vi "ValveMonitoring.vi"() -> ()   [LabVIEW 2020]
uses:
  Control/MainProgramState.ctl
  <vilib>/DAQmx/read.llb/DAQmx Read (Analog 1D DBL NChan 1Samp).vi
  <vilib>/DAQmx/create/channels.llb/DAQmx Create Channel (AI-Voltage-Basic).vi
  <vilib>/DAQmx/miscellaneous.llb/DAQmx Fill In Error Info.vi
  <resource>/objmgr/daqmx.rc
panel:
  out "RemainTime":dbl(slide) scale=0.0..1.0
  in  "TermiateTime(min)":dbl=60.0 format="%.1f"
  out "FlowRate(Average)":dbl format="%.3f"
  out "ProgramState":T1
  out "Active":bool
  in  "Set":bool
  out "TestTimer(sec)":dbl format="%.1f"
  out "SystemTimer(sec)":dbl format="%.1f"
  out "FlowRate":dbl format="%.3f"
  out "Pressure":dbl format="%.1f"
  out "TestTimer(min)":dbl
  out "FlowRateLowWarning":bool
  in  "FlowRateUpperLimit(LPM)":dbl=1.0 format="%.3f"
  in  "PressureLowerLimit(bar)":dbl=5.0 format="%.1f"
  out "PressureLowWarning":bool
  in  "Reset":bool
  out "SystemTimer(min)":dbl
  in  "FileName":string="Test"
  in  "Stop":bool
  in  "Pause":bool
  in  "Start":bool
  out "StopSignal":bool
  out "appended array":dbl[](array[numeric])
  out "FlowRate":cluster{dbl[], dbl[]}(graph)
  out "Pressure":cluster{dbl[], dbl[]}(graph)
  # "Test Setting"
  # "<- Logging Fine Name"
  # "Program State"
  # "System Timer"
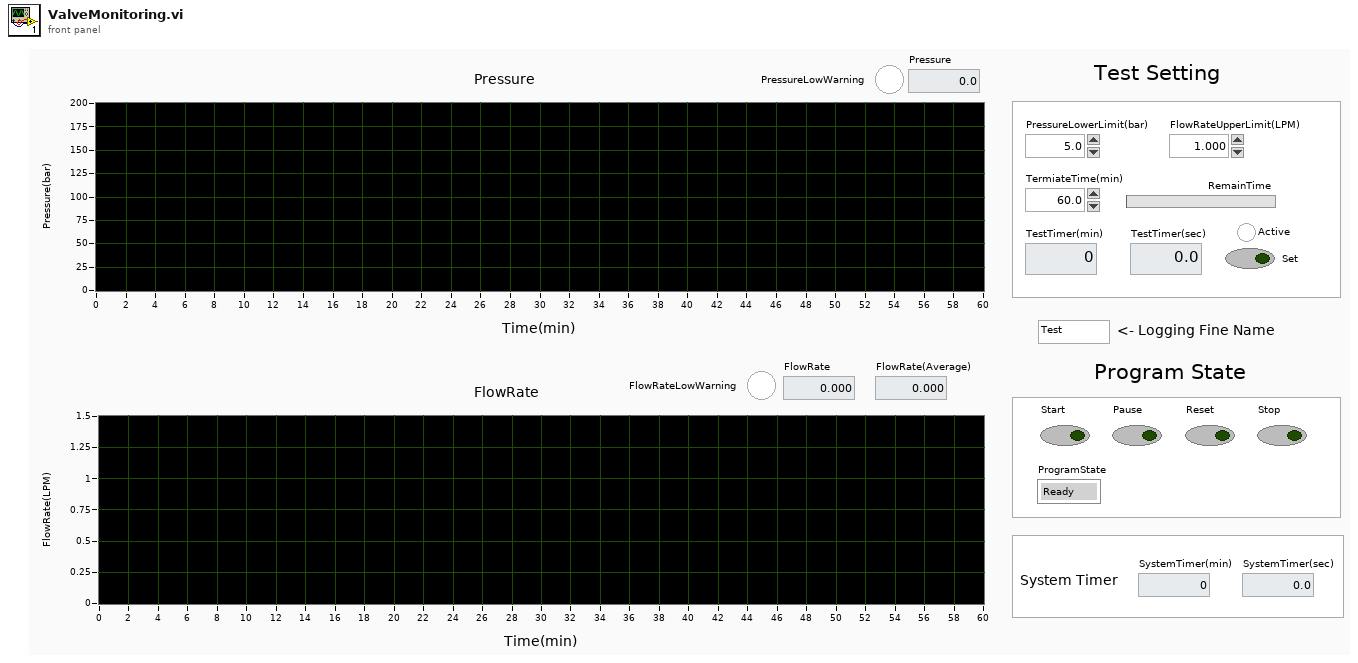
[diagram p1: front panel]
types:
  T1 = typedef "MainProgramState.ctl" = enum16{"Ready", "Run", "Pause", "Reset", "Stop"}
  T2 = cluster{"State":T1, "MainTimer(sec)":dbl, "TestTimer(sec)":dbl}
  T3 = enum16{"open", "replace", "create", "open or create", "replace or create", "replace or create with confirmation"}
  T4 = cluster{"getFlowRate":dbl, "getPressure":dbl, "setFlowRate":dbl, "setPressure":dbl}
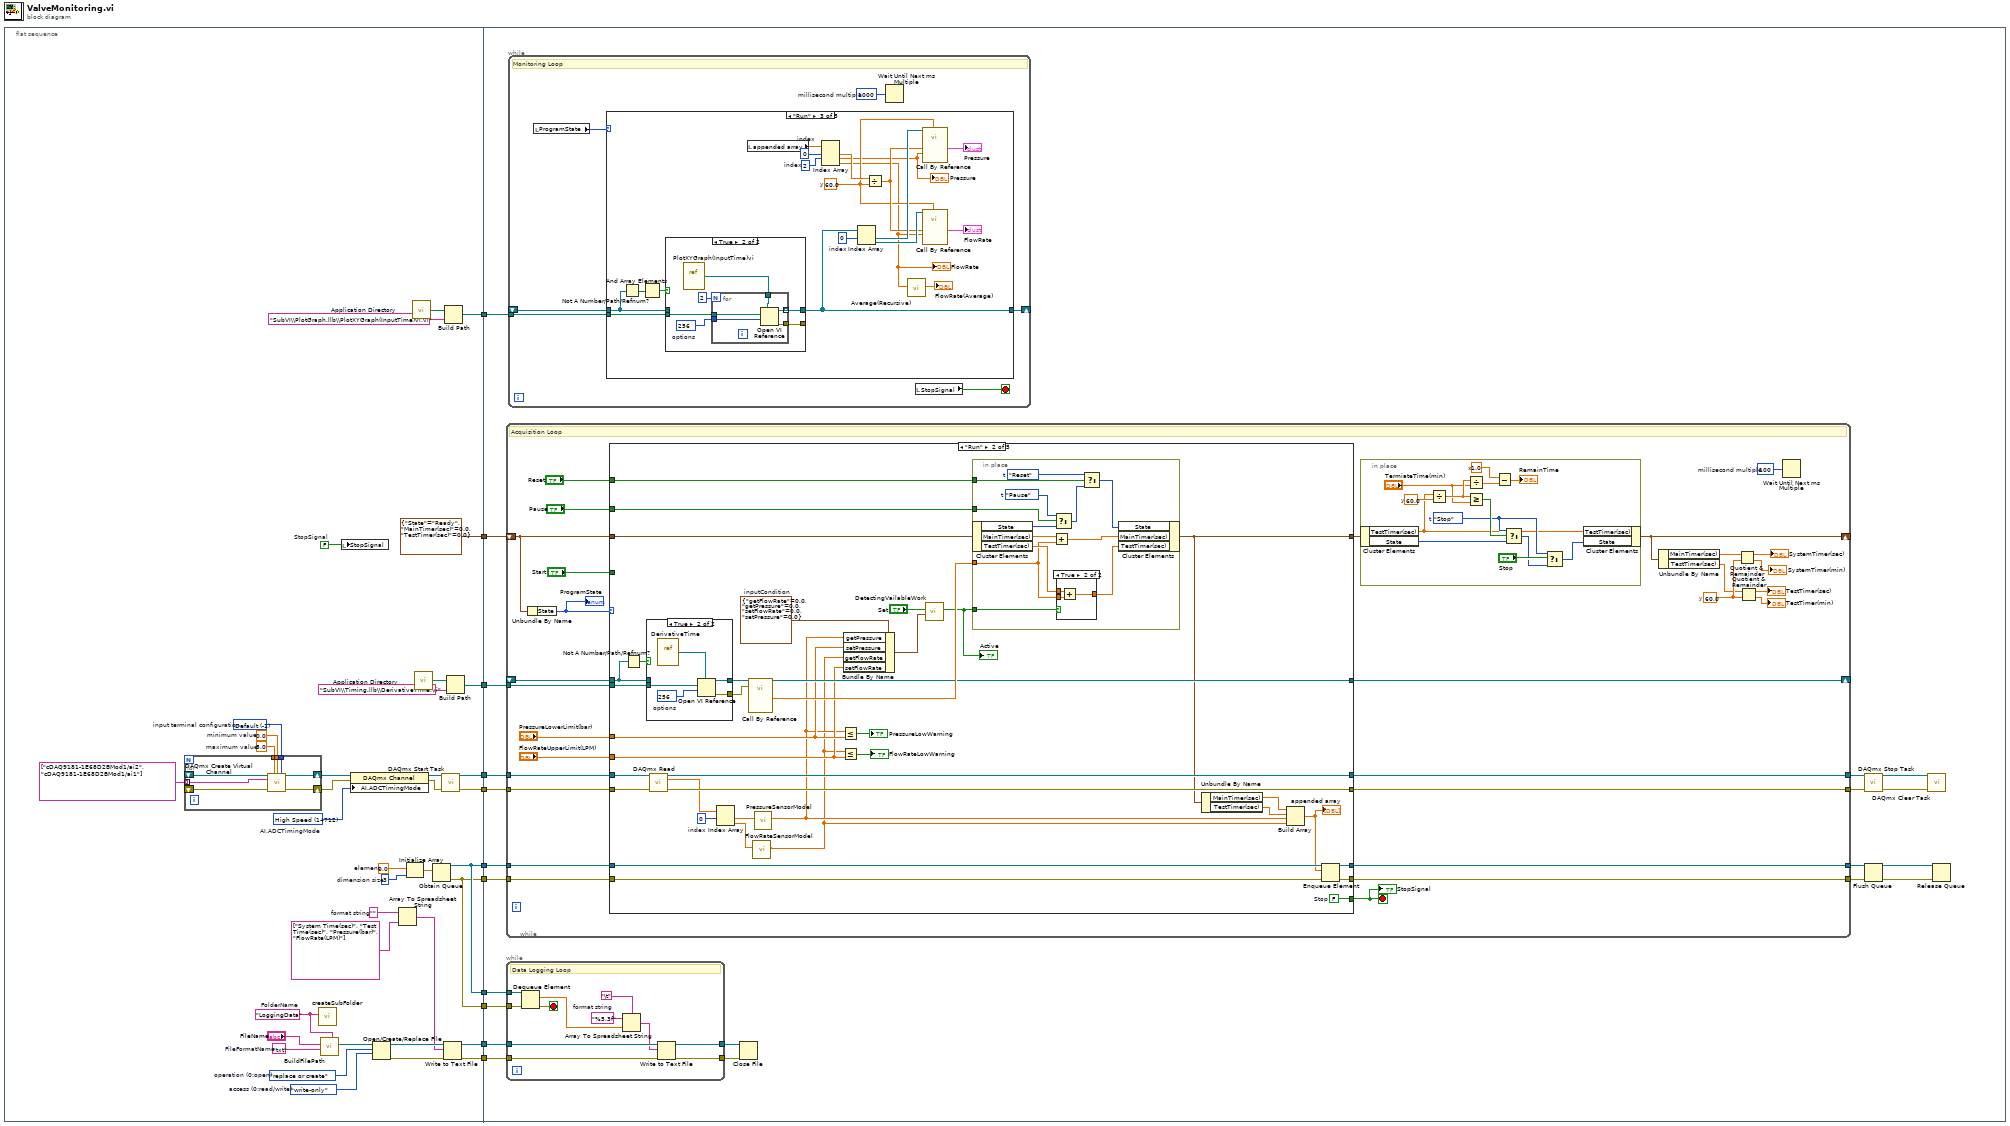
[diagram p0: block diagram]
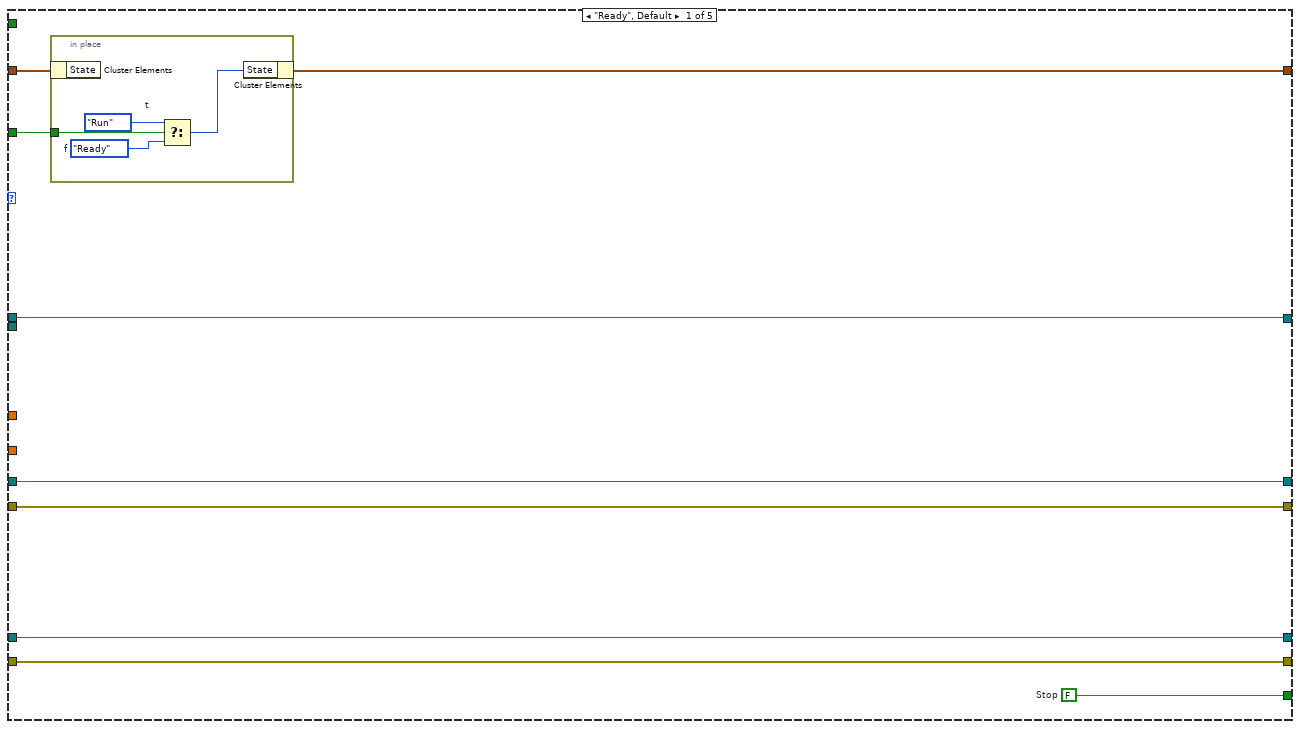
[diagram p2: hidden frame]
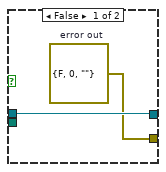
[diagram p3: hidden frame]
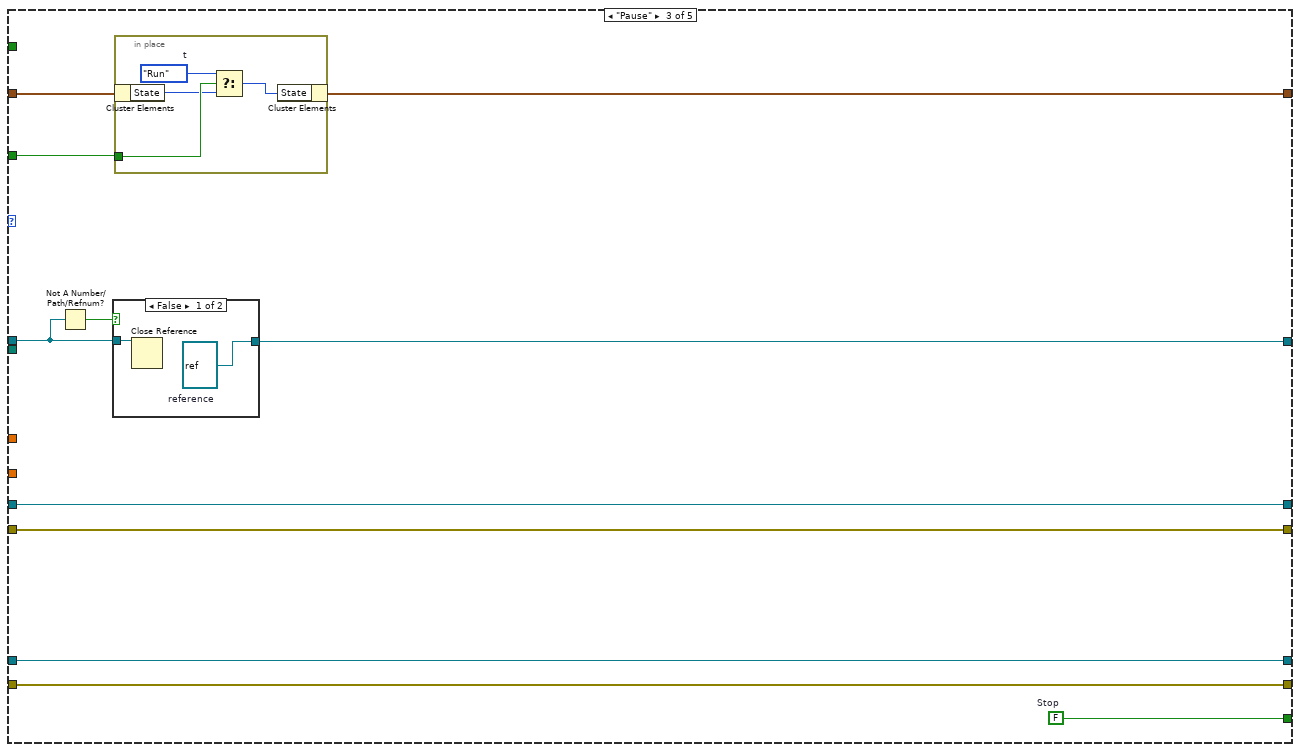
[diagram p5: hidden frame]
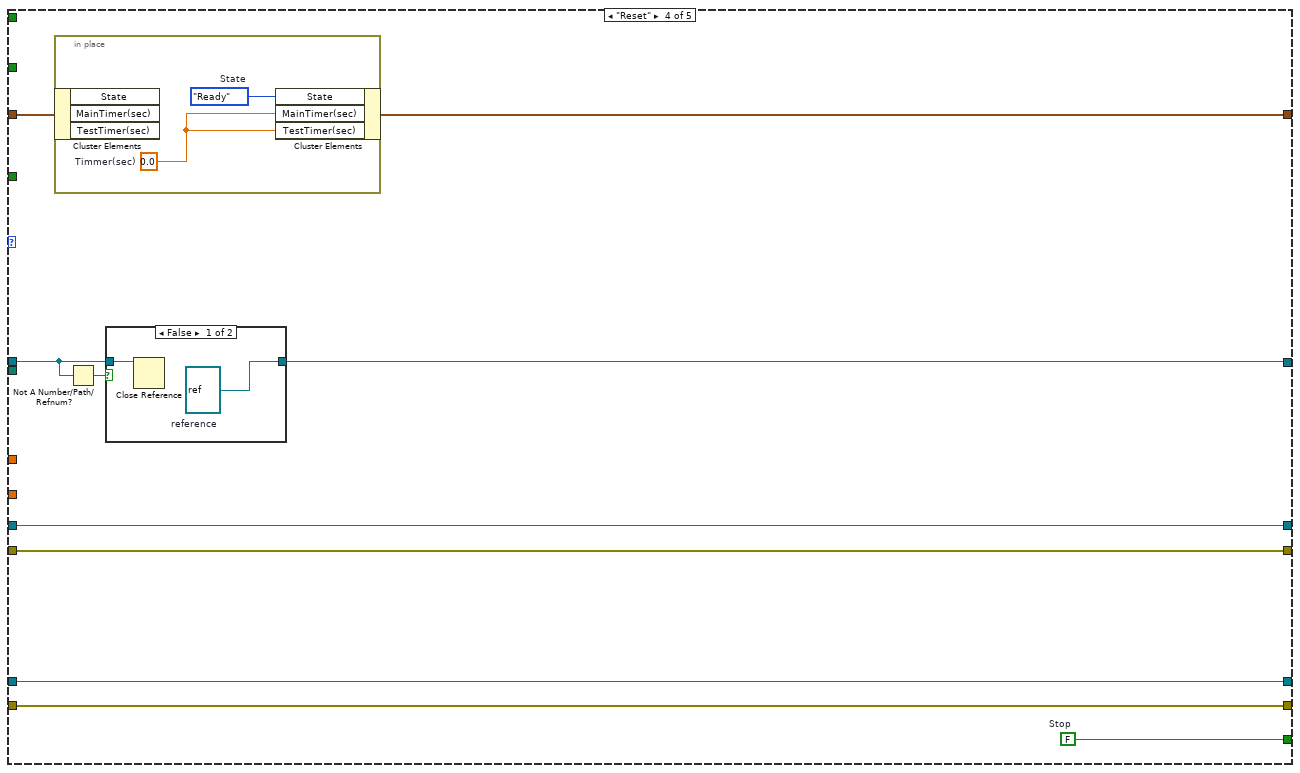
[diagram p7: hidden frame]
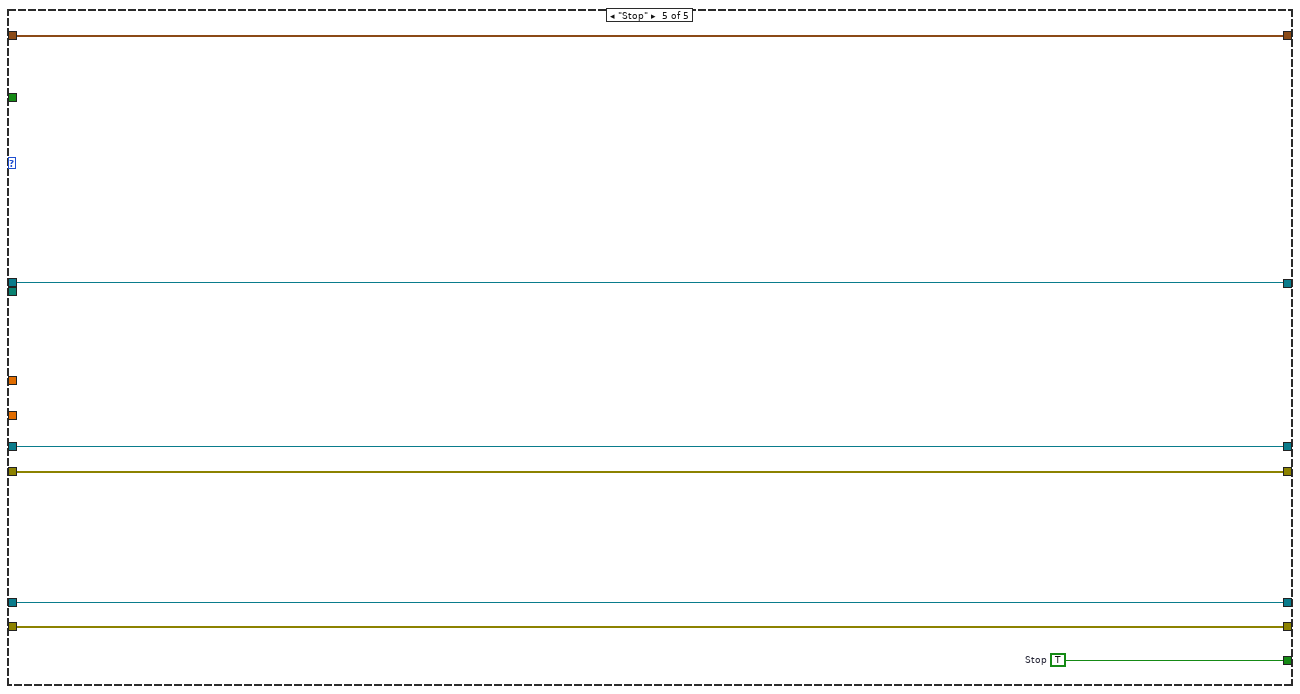
[diagram p9: hidden frame]
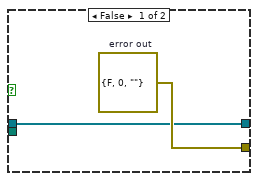
[diagram p12: hidden frame]
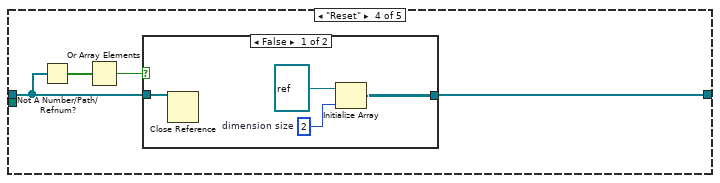
[diagram p13: hidden frame]
diagram:
  n1 = flat-sequence {
    tunnel: [w36] -> w11
    tunnel: [w35] -> w10
    tunnel: [w43] -> w9
    tunnel: [w42] -> w8
    tunnel: [w43] -> w7
    tunnel: [w42] -> w6
    tunnel: [w32] -> w5
    tunnel: [w31] -> w4
    tunnel: [T2 {"State"=enum."Ready", "MainTimer(sec)"=0.0, "TestTimer(sec)"=0.0}] -> w3
    tunnel: [w16] -> w2
    tunnel: [w12] -> w1
    tunnel: w11 -> [w77]
    tunnel: w10 -> [w72]
    tunnel: w9 -> [w71]
    tunnel: w8 -> [w70]
    tunnel: w7 -> [w65]
    tunnel: w6 -> [w64]
    tunnel: w5 -> [w63]
    tunnel: w4 -> [w62]
    tunnel: w3 -> [w59]
    tunnel: w2 -> [w58]
    tunnel: w1 -> [w57]
    frame #0 {
      w18 = FALSE  # StopSignal
      w19 = 14712 items=["Automatic"=16097, "High Resolution"=10195, "High Speed"=14712, "Best 50 Hz Rejection"=14713, "Best 60 Hz Rejection"=14714, "Custom"=10137]  # AI.ADCTimingMode
      w25 = "txt"  # FileFormatName
      w28 = ""  # format string
      w37 = enum16{"read/write", "read-only", "write-only"}."write-only"  # access (0:read/write)
      w38 = T3."replace or create"  # operation (0:open)
      w40 = "LoggingData"  # FolderName
      w41 = -1 items=["Default"=-1, "RSE"=10083, "NRSE"=10078, "Differential"=10106, "Pseudodifferential"=12529]  # input terminal configuration
      w45 = 3  # dimension size
      w46 = 0.0  # element
      w47 = 0.0  # minimum value
      w48 = 5.0  # maximum value
      n2 = for {
        tunnel: w48 -> [w56]
        tunnel: w47 -> [w55]
        tunnel: w41 -> [w54]
        shift-right: [w53] -> w24
        shift-left: _ -> [w52]
        tunnel: tag[] ["cDAQ9181-1E68D2BMod1/ai2", "cDAQ9181-1E68D2BMod1/ai1"] -> [w51] mode=indexing
        shift-right: [w50] -> w21
        shift-left: _ -> [w49]
        n3 = call-poly <vilib>:"DAQmx Create Virtual Channel.vi"("task in"=w52, "maximum value"=w56, "minimum value"=w55, "input terminal configuration"=w54, "physical channels"=w51, "error in"=w49) -> ("task out"=w53:refnum<k21>, "error out"=w50:errorcluster)  [unwired: 8 in]
      }
      n4 = call "createSubFolder.vi"("FolderName"=w40) -> ()  [unwired: 10 in, 1 out]
      n5 = call "BuildFilePath.vi"("SubFolderName"=w40, "FileFormatName"=w25, "FileName"="FileName") -> ("appended path"=w39:path)  [unwired: 8 in]
      n6 = local write "StopSignal"(w18) -> ()
      n7 = property class="DAQmx Channel"(reference=w24, error in=w21, "AI.ADCTimingMode"=w19) -> (reference out=w22:refnum<k21>, error out=w20:errorcluster)
      n8 = Open/Create/Replace File(file path (use dialog)=w39, operation (0:open)=w38, access (0:read/write)=w37) -> (refnum out=w34:refnum<file>, error out=w33:errorcluster)  [unwired: 3 in, 1 out]
      n9 = Array To Spreadsheet String(array=string[] ["System Time(sec)", "Test Time(sec)", "Pressure(bar)", "FlowRate(LPM)"], 3:w28) -> (spreadsheet string=w29:string)  [unwired: 1 in]
      n10 = Initialize Array "Initialize Array"(w46, w45) -> (w44:dbl[])
      n11 = call <vilib>:"Application Directory.vi"() -> ("Application Directory"=w14:path)
      n12 = call <vilib>:"Application Directory.vi"() -> ("Application Directory"=w15:path)
      n13 = Obtain Queue(element data type=w44) -> (queue out=w43:refnum<queue>, error out=w42:errorcluster)  [unwired: 4 in, 1 out]
      n14 = call <vilib>:"DAQmx Start Task.vi"("task/channels in"=w22, "error in"=w20) -> ("task out"=w36:refnum<k21>, "error out"=w35:errorcluster)  [unwired: 12 in]
      n15 = Write to Text File(file (use dialog)=w34, text=w29, error in=w33) -> (refnum out=w32:refnum<file>, error out=w31:errorcluster)  [unwired: 1 in, 1 out]
      n16 = Build Path(base path=w14, name or relative path="SubVI\\PlotGraph.llb\\PlotXYGraph(InputTime)vi.vi") -> (appended path=w12:path)
      n17 = Build Path(base path=w15, name or relative path="SubVI\\Timing.llb\\DerivativeTime.vi") -> (appended path=w16:path)
    }
    frame #1 {
      n18 = while {
        tunnel: w77 -> [w117]
        tunnel: [w116] -> w76
        tunnel: [w115] -> w74
        tunnel: w72 -> [w114]
        tunnel: w71 -> [w113]
        tunnel: w70 -> [w112]
        tunnel: [w111] -> w69
        tunnel: [w110] -> w68
        shift-right: [w102] -> _
        shift-left: w59 -> [w104]
        tunnel: w58 -> [w101]
        shift-right: [w100] -> _
        shift-left: _ -> [w99]
        stop <- w106 stop-if-true
        w91 = 60.0  # y
        w109 = u32 100  # millisecond multiple
        # "Acquisition Loop"
        n19 = Unbundle By Name(w104) -> ("State"=w105:T1)
        "ProgramState" <- w105
        n20 = case shown="\"Run\"" w105 {
          tunnel: w117 -> [w126 w167 w202 w217 w228]
          tunnel: [w126 w166 w202 w217 w228] -> w116
          tunnel: [w125 w165 w201 w216 w227] -> w115
          tunnel: w114 -> [w125 w164 w201 w216 w227]
          tunnel: w113 -> [w124 w163 w200 w215 w230]
          tunnel: w112 -> [w123 w162 w199 w214 w229]
          tunnel: [w124 w161 w200 w215 w230] -> w111
          tunnel: [w123 w160 w199 w214 w229] -> w110
          tunnel: "Start" -> [w119 _ w195 _ _]
          tunnel: "Pause" -> [_ w157 _ _ _]
          tunnel: [w122 w159 w198 w213 w231] -> w106
          tunnel: [w120 w133 w196 w218 w226] -> w103
          tunnel: w104 -> [w121 w153 w197 w219 w226]
          tunnel: w101 -> [_ w154 _ _ _]
          tunnel: [w118 w150 w192 w210 w225] -> w100
          tunnel: w99 -> [w118 w149 w193 w211 w225]
          tunnel: "Reset" -> [_ w144 _ _ _]
          tunnel: "PressureLowerLimit(bar)" -> [_ w141 _ _ _]
          tunnel: "FlowRateUpperLimit(LPM)" -> [_ w140 _ _ _]
          frame "Ready", Default {
            w122 = FALSE  # Stop
            n21 = in-place {
              in-place-border: w119 -> [w128]
              w130 = MainProgramState."Ready"  # f
              w129 = MainProgramState."Run"  # t
              n22 = in-place-cluster #1(w121) -> ()  [unwired: 1 out]
              n23 = Select(t=w129, s=w128, f=w130) -> (s? t:f=w127:T1)
              n24 = in-place-cluster #1("State"=w127) -> (w120:T2)
            }
          }
          frame "Run" {
            w139 = T4 {"getFlowRate"=0.0, "getPressure"=0.0, "setFlowRate"=0.0, "setPressure"=0.0}  # inputCondition
            w147 = 0  # index
            w159 = FALSE  # Stop
            n25 = Not A Number/Path/Refnum?(number/path/refnum=w149) -> (NaN/Path/Refnum?=w155:bool)
            n26 = case shown="True" w155 {
              tunnel: w154 -> [_ w173]
              tunnel: [w169 w171] -> w152
              tunnel: [w168 w170] -> w151
              tunnel: w149 -> [w169 _]
              frame False {
                w168 = errorcluster {"status"=FALSE, "code"=0, "source"=""}  # error out
              }
              frame True {
                w174 = 256  # options
                n27 = vi-ref "DerivativeTime.vi"() -> (w172:refnum<vi>)
                n28 = Open VI Reference(type specifier VI Refnum (for type only)=w172, vi path=w173, options=w174) -> (vi reference=w171:refnum<vi>, error out=w170:errorcluster)  [unwired: 3 in]
              }
            }
            n29 = call-poly <vilib>:"DAQmx Read.vi"("task/channels in"=w167, "error in"=w164) -> ("task out"=w166:refnum<k21>, "data"=w148:dbl[], "error out"=w165:errorcluster)  [unwired: 11 in]
            n30 = Index Array "Index Array"(array=w148, index #1=w147) -> (element #1=w145:dbl, element #2=w146:dbl)  [unwired: 1 in]
            n31 = call-by-ref "Call By Reference"(reference=w152, error in=w151) -> (reference out=w150:refnum<vi>, "Time(sec)"=w156:dbl)  [unwired: 11 in, 1 out]
            n32 = call "FlowRateSensorModel.vi"("inputSignal(V)"=w146) -> ("FlowRate(LPM)"=w134:dbl)  [unwired: 10 in]
            n33 = call "PressureSensorModel.vi"("inputSignal(V)"=w145) -> ("Pressure(bar)"=w135:dbl)  [unwired: 10 in]
            n34 = Less Or Equal?(x=w135, y=w141) -> (x <= y?=→"PressureLowWarning":bool)
            n35 = Less Or Equal?(x=w134, y=w140) -> (x <= y?=→"FlowRateLowWarning":bool)
            n36 = Bundle By Name(cluster=w139, "getPressure"=w135, "setPressure"=w141, "getFlowRate"=w134, "setFlowRate"=w140) -> (w138:T4)
            n37 = call "DetectingVailableWork.vi"("inputCondition"=w138, "Reset"="Set") -> ("Progressing"=w137:bool)  [unwired: 9 in]
            "Active" <- w137
            n38 = in-place {
              in-place-border: w156 -> [w181]
              in-place-border: w157 -> [w184]
              in-place-border: w144 -> [w179]
              in-place-border: w137 -> [w175]
              w177 = MainProgramState."Reset"  # t
              w183 = MainProgramState."Pause"  # t
              n39 = in-place-cluster #2(w153) -> ("State"=w185:T1, "MainTimer(sec)"=w187:dbl, "TestTimer(sec)"=w182:dbl)
              n40 = Add(x=w187, y=w181) -> (x+y=w186:dbl)
              n41 = Select(t=w183, s=w184, f=w185) -> (s? t:f=w180:T1)
              n42 = case shown="True" w175 {
                tunnel: w182 -> [w188 w191]
                tunnel: w181 -> [_ w190]
                tunnel: [w188 w189] -> w176
                frame False {
                }
                frame True {
                  n43 = Add(x=w191, y=w190) -> (x+y=w189:dbl)
                }
              }
              n44 = Select(t=w177, s=w179, f=w180) -> (s? t:f=w178:T1)
              n45 = in-place-cluster #2("State"=w178, "MainTimer(sec)"=w186, "TestTimer(sec)"=w176) -> (w133:T2)
            }
            n46 = Unbundle By Name(w133) -> ("MainTimer(sec)"=w132:dbl, "TestTimer(sec)"=w131:dbl)
            n47 = Build Array "Build Array"(w132, w131, w135, w134) -> (w158:dbl[])
            "appended array" <- w158
            n48 = Enqueue Element(queue=w163, element=w158, error in (no error)=w162) -> (queue out=w161:refnum<queue>, error out=w160:errorcluster)  [unwired: 1 in, 1 out]
          }
          frame "Pause" {
            w198 = FALSE  # Stop
            n49 = Not A Number/Path/Refnum?(number/path/refnum=w193) -> (NaN/Path/Refnum?=w194:bool)
            n50 = case shown="False" w194 {
              tunnel: w193 -> [w204 w205]
              tunnel: [w203 w205] -> w192
              frame False {
                w203 = refnum<vi> refnum  # reference
                n51 = Close Reference(reference=w204) -> ()  [unwired: 1 in, 1 out]
              }
              frame True {
              }
            }
            n52 = in-place {
              in-place-border: w195 -> [w209]
              w206 = MainProgramState."Run"  # t
              n53 = in-place-cluster #3(w197) -> ("State"=w208:T1)
              n54 = Select(t=w206, s=w209, f=w208) -> (s? t:f=w207:T1)
              n55 = in-place-cluster #3("State"=w207) -> (w196:T2)
            }
          }
          frame "Reset" {
            w213 = FALSE  # Stop
            n56 = in-place {
              w224 = MainProgramState."Ready"  # State
              w223 = 0.0  # Timmer(sec)
              n57 = in-place-cluster #4(w219) -> ()  [unwired: 3 out]
              n58 = in-place-cluster #4("State"=w224, "MainTimer(sec)"=w223, "TestTimer(sec)"=w223) -> (w218:T2)
            }
            n59 = Not A Number/Path/Refnum?(number/path/refnum=w211) -> (NaN/Path/Refnum?=w212:bool)
            n60 = case shown="False" w212 {
              tunnel: w211 -> [w221 w222]
              tunnel: [w220 w222] -> w210
              frame False {
                w220 = refnum<vi> refnum  # reference
                n61 = Close Reference(reference=w221) -> ()  [unwired: 1 in, 1 out]
              }
              frame True {
              }
            }
          }
          frame "Stop" {
            w231 = TRUE  # Stop
          }
        }
        "StopSignal" <- w106
        n62 = in-place {
          w233 = 1.0  # x
          w243 = 60.0  # y
          w239 = MainProgramState."Stop"  # t
          n63 = in-place-cluster #5(w103) -> ("TestTimer(sec)"=w237:dbl, "State"=w241:T1)
          n64 = Divide(x=w237, y=w243) -> (x/y=w236:dbl)
          n65 = Divide(x=w236, y="TermiateTime(min)") -> (x/y=w234:dbl)
          n66 = Greater Or Equal?(x=w236, y="TermiateTime(min)") -> (x >= y?=w242:bool)
          n67 = Subtract(x=w233, y=w234) -> (x-y=→"RemainTime":dbl)
          n68 = Select(t=w239, s=w242, f=w241) -> (s? t:f=w240:T1)
          n69 = Select(t=w239, s="Stop", f=w240) -> (s? t:f=w238:T1)
          n70 = in-place-cluster #5("TestTimer(sec)"=w237, "State"=w238) -> (w102:T2)
        }
        n71 = Unbundle By Name(w102) -> ("MainTimer(sec)"=w95:dbl, "TestTimer(sec)"=w90:dbl)
        n72 = Quotient & Remainder(x=w95, y=w91) -> (x-y*floor(x/y)=→"SystemTimer(sec)":dbl, floor(x/y)=→"SystemTimer(min)":dbl)
        n73 = Quotient & Remainder(x=w90, y=w91) -> (x-y*floor(x/y)=→"TestTimer(sec)":dbl, floor(x/y)=→"TestTimer(min)":dbl)
        n74 = Wait Until Next ms Multiple(millisecond multiple=w109) -> ()  [unwired: 1 out]
      }
      n75 = while {
        tunnel: w65 -> [w88]
        tunnel: w64 -> [w87]
        tunnel: w63 -> [w85]
        tunnel: w62 -> [w80]
        tunnel: [w79] -> w61
        tunnel: [w78] -> w60
        stop <- w86 stop-if-true
        w83 = "%5.3f"  # format string
        # "Data Logging Loop"
        n76 = Dequeue Element(queue=w88, error in (no error)=w87) -> (element=w82:dbl[], error out=w86:errorcluster)  [unwired: 1 in, 2 out]
        n77 = Array To Spreadsheet String(delimiter (Tab)="\t", array=w82, 3:w83) -> (spreadsheet string=w81:string)
        n78 = Write to Text File(file (use dialog)=w85, text=w81, error in=w80) -> (refnum out=w79:refnum<file>, error out=w78:errorcluster)  [unwired: 1 in, 1 out]
      }
      n79 = while {
        tunnel: w57 -> [w247]
        shift-right: [w246] -> _
        shift-left: _ -> [w245]
        stop <- w249 stop-if-true
        w250 = u32 1000  # millisecond multiple
        # "Monitoring Loop"
        n80 = local read "ProgramState"() -> (w248:T1)
        n81 = case shown="\"Run\"" w248 {
          tunnel: w247 -> [_ _ w268 _ _]
          tunnel: [w251 w252 w266 w285 w294] -> w246
          tunnel: w245 -> [w251 w252 w263 w287 w294]
          frame "Ready", Default {
          }
          frame "Pause" {
          }
          frame "Run" {
            w255 = 2  # index
            w267 = 0  # index
            w257 = 60.0  # y
            w270 = 0  # index
            n82 = Not A Number/Path/Refnum?(number/path/refnum=w263) -> (NaN/Path/Refnum?=w265:bool[])
            n83 = And Array Elements(Boolean array=w265) -> (logical AND=w264:bool)
            n84 = case shown="True" w264 {
              tunnel: w268 -> [_ w278]
              tunnel: [w272 w276] -> w266
              tunnel: [w273 w275] -> _
              tunnel: w263 -> [w272 _]
              frame False {
                w273 = errorcluster {"status"=FALSE, "code"=0, "source"=""}  # error out
              }
              frame True {
                w279 = 256  # options
                n85 = vi-ref "PlotXYGraph(InputTime)vi.vi"() -> (w277:refnum<vi>)
                n86 = for {
                  N: 2 -> [_]
                  tunnel: w279 -> [w284]
                  tunnel: w278 -> [w283]
                  tunnel: [w280] -> w275
                  tunnel: w277 -> [w282]
                  tunnel: [w281] -> w276 mode=indexing
                  n87 = Open VI Reference(type specifier VI Refnum (for type only)=w282, vi path=w283, options=w284) -> (vi reference=w281:refnum<vi>, error out=w280:errorcluster)  [unwired: 3 in]
                }
              }
            }
            n88 = local read "appended array"() -> (w271:dbl[])
            n89 = Index Array "Index Array"(array=w271, index #1=w270, index #2=w255) -> (element #1=w269:dbl, element #2=w256:dbl, element #3=w254:dbl)  [unwired: 1 in]
            "Pressure" <- w256
            "FlowRate" <- w254
            n90 = Index Array(array=w266, index #1=w267) -> (element #1=w262:refnum<vi>, element #2=w259:refnum<vi>)  [unwired: 1 in]
            n91 = Divide(x=w269, y=w257) -> (x/y=w258:dbl)
            n92 = call "Average(Recursive).vi"("DataInput"=w254) -> ("Average"=→"FlowRate(Average)":dbl)  [unwired: 10 in]
            n93 = call-by-ref "Call By Reference"(reference=w262, "Length(sec)"=w257, "inputData"=w256, "inputTime(sec)"=w258) -> ("outputGraph"=→"Pressure":cluster{"Time":dbl[], "Data":dbl[]})  [unwired: 9 in, 2 out]
            n94 = call-by-ref "Call By Reference"(reference=w259, "Length(sec)"=w257, "inputData"=w254, "inputTime(sec)"=w258) -> ("outputGraph"=→"FlowRate":cluster{"Time":dbl[], "Data":dbl[]})  [unwired: 9 in, 2 out]
          }
          frame "Reset" {
            n95 = Not A Number/Path/Refnum?(number/path/refnum=w287) -> (NaN/Path/Refnum?=w288:bool[])
            n96 = Or Array Elements(Boolean array=w288) -> (logical OR=w286:bool)
            n97 = case shown="False" w286 {
              tunnel: w287 -> [w292 w293]
              tunnel: [w289 w293] -> w285
              frame False {
                w290 = 2  # dimension size
                n98 = Close Reference(reference=w292) -> ()  [unwired: 1 in, 1 out]
                n99 = Initialize Array "Initialize Array"(refnum<vi> refnum, w290) -> (w289:refnum<vi>[])
              }
              frame True {
              }
            }
          }
          frame "Stop" {
          }
        }
        n100 = Wait Until Next ms Multiple(millisecond multiple=w250) -> ()  [unwired: 1 out]
        n101 = local read "StopSignal"() -> (w249:bool)
      }
      n102 = Close File(refnum=w61, error in=w60) -> ()  [unwired: 2 out]
      n103 = call <vilib>:"DAQmx Stop Task.vi"("task/channels in"=w76, "error in"=w74) -> ("task out"=w75:refnum<k21>, "error out"=w73:errorcluster)  [unwired: 12 in]
      n104 = Flush Queue(queue=w69, error in (no error)=w68) -> (queue out=w67:refnum<queue>, error out=w66:errorcluster)  [unwired: 1 out]
      n105 = call <vilib>:"DAQmx Clear Task.vi"("task in"=w75, "error in"=w73) -> ()  [unwired: 13 in, 1 out]
      n106 = Release Queue(queue=w67, error in (no error)=w66) -> ()  [unwired: 1 in, 3 out]
    }
  }
